vi "xijk_image_interpolate.vi"(8 "error in":errorcluster, 11 "array in":dbl[][](array[numeric])=[[395.7325746799431, 6.581740976645436], [444.80796586059745, 1.6985138004246285], [470.41251778093886, 0.6369426751592357], [491.74964438122333, 1.2738853503184715], [502.4182076813656, 4.883227176220807], [510.9530583214794, 1.910828025477707], [532.2901849217639, 1.910828025477707], [557.8947368421052, 4.45859872611465], [562.1621621621621, 1.6985138004246285], [606.9701280227596, -0.21231422505307856], [641.1095305832148, 1.48619957537155], [662.4466571834993, 2.547770700636943], [688.0512091038406, 2.9723991507431], [739.2603129445234, 24.840764331210192], [775.5334281650071, 52.01698513800425], [788.3357041251777, 76.64543524416136]]) -> (0 "error out":errorcluster, 3 "array out":dbl[][](array[numeric]))   [LabVIEW 2010]
uses:
  <vilib>/gmath/NI_Gmath.lvlib
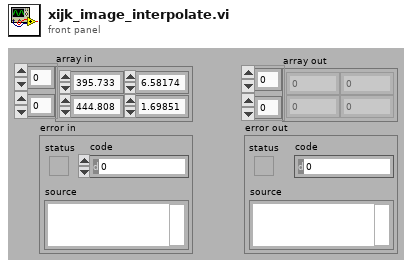
[diagram p1: front panel]
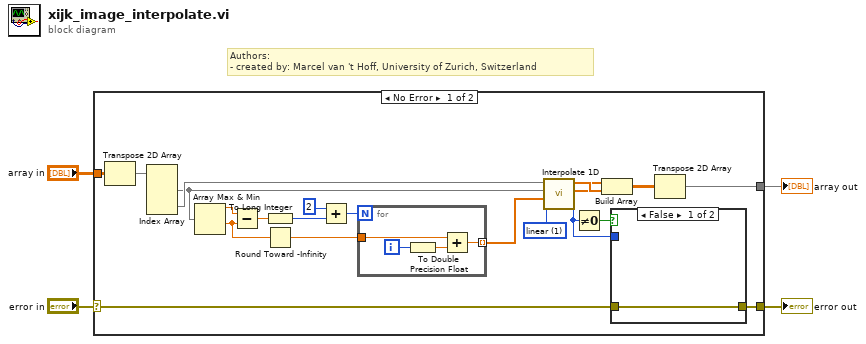
[diagram p0: block diagram]
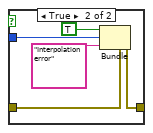
[diagram p2: hidden frame]
diagram:
  # "Authors: \n- created by: Marcel van 't Hoff, University of Zurich, Switzerland"
  n1 = case shown="No Error" "error in" {
    selector: "error in" -> [w12 w36]
    tunnel: "array in" -> [w25 _]
    tunnel: [w9 w36] -> w2
    tunnel: [w7 _] -> w1
    frame No Error {
      w22 = 1 items=["nearest", "linear", "spline", "cubic Hermite", "Lagrange"] ("method")
      n2 = Transpose 2D Array(2D array=w25) -> (transposed array=w24:dbl[][])
      n3 = Index Array(array=w24) -> (element #1=w21:dbl[], element #2=w23:dbl[])  [unwired: 4 in]
      n4 = Array Max & Min(array=w21) -> (max value=w20:dbl, min value=w17:dbl)  [unwired: 2 out]
      n5 = Subtract(x=w20, y=w17) -> (x-y=w19:dbl)
      n6 = To Long Integer(number=w19) -> (32bit integer=w18:i32)
      n7 = Round Toward -Infinity(1:w17) -> (0:w16:dbl)
      n8 = Add(x=2, y=w18) -> (x+y=w15:i32)
      n9 = for {
        N: w15 -> [_]
        tunnel: w16 -> [w34]
        tunnel: [w33] -> w13 mode=indexing
        i -> [w35]
        n10 = To Double Precision Float(number=w35) -> (double precision float=w32:dbl)
        n11 = Add(x=w34, y=w32) -> (x+y=w33:dbl)
      }
      n12 = call <vilib>:"Interpolate 1D.vi"("method"=w22, "xi"=w13, "X"=w21, "Y"=w23) -> ("error"=w10:i32, "xi used"=w5:dbl[], "yi"=w6:dbl[])  [unwired: 5 in]
      n13 = Not Equal To 0?(x=w10) -> (x != 0?=w11:bool)
      n14 = Build Array(w5, w6) -> (w8:dbl[][])
      n15 = case shown="False" w11 {
        tunnel: w12 -> [w26 w31]
        tunnel: w10 -> [_ w29]
        tunnel: [w26 w27] -> w9
        frame False {
        }
        frame True {
          n16 = Bundle(cluster=w31, "status"=TRUE, "code"=w29, "source"="Interpolation error") -> (w27:errorcluster)
        }
      }
      n17 = Transpose 2D Array(2D array=w8) -> (transposed array=w7:dbl[][])
    }
    frame Error {
    }
  }
  "error out" <- w2
  "array out" <- w1
